vi "sing_mess.vi"(7 "Timeout(默认:5ms)":i32=5, 8 "error in":errorcluster, 9 "COM通道":u32=1, 10 "索引":i32, 11 "VISA资源名称":refnum<visa-resource-name>) -> (0 "error out 2":errorcluster, 1 "timeout":bool, 3 "VISAout":refnum<visa-resource-name>)   [LabVIEW 2012]
uses:
  com/TONGXUN/write32.vi
  com/TONGXUN/write8.vi
  <vilib>/GPower/VIRegister/VIRegister.lvlib
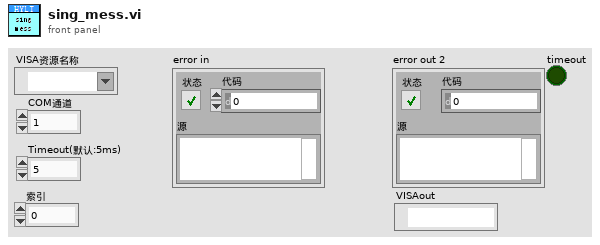
[diagram p1: front panel]
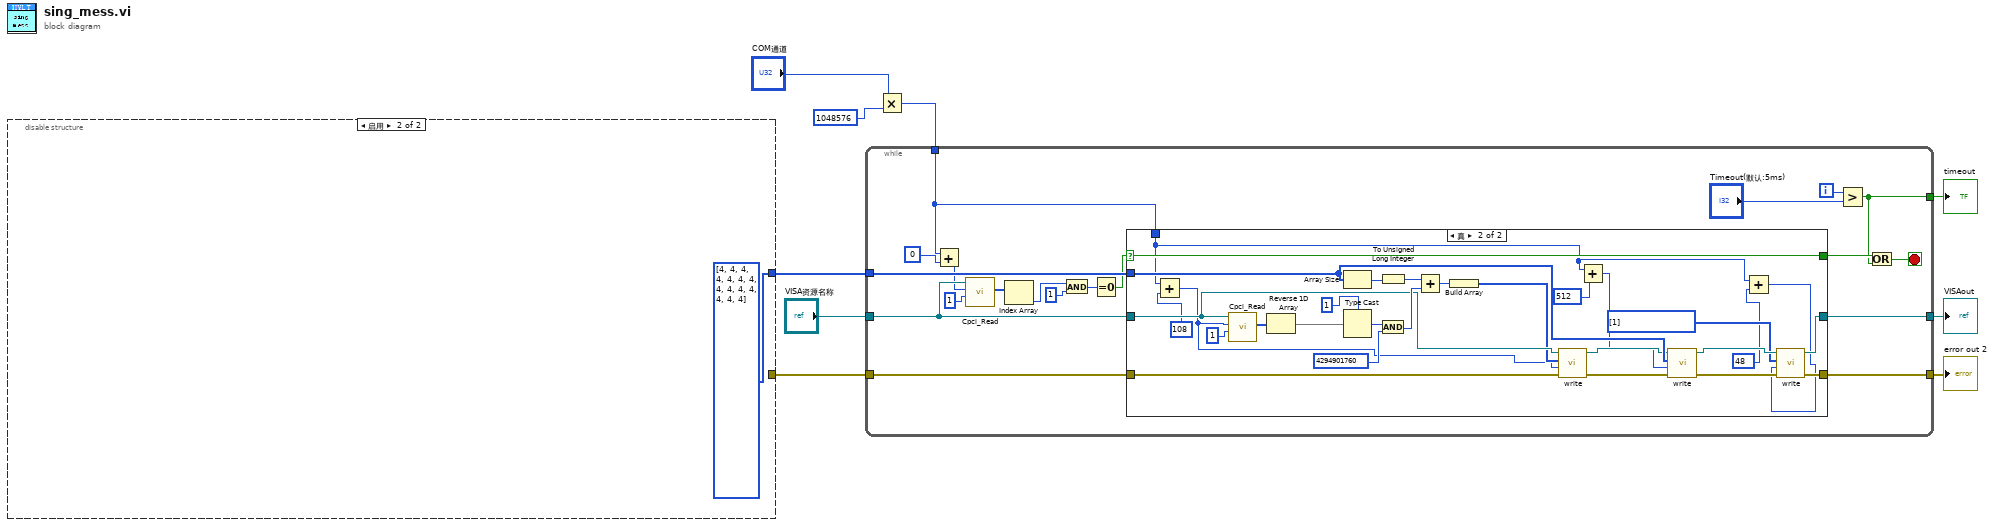
[diagram p0: block diagram]
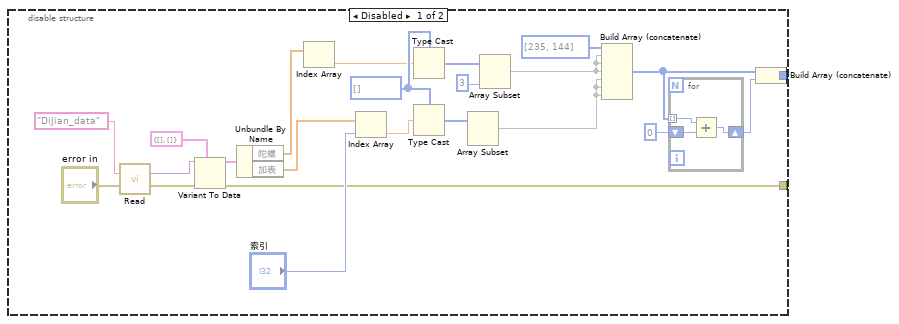
[diagram p2: hidden frame]
diagram:
  n1 = disable-structure shown="启用" {
    disable-tunnel: [w13 u8[] [4, 4, 4, 4, 4, 4, 4, 4, 4, 4, 4, 4, 4, 4]] -> w5
    disable-tunnel: [w11 _] -> w4
    frame Disabled {
      w32 = u8[] []
      n2 = call <vilib>:"Read.vi"("Register name"="DiJian_data", "Error in"="error in") -> ("Register value"=w22:variant, "Error out"=w12:errorcluster)  [unwired: 10 in, 2 out]
      n3 = Variant To Data(error in=w12, type=cluster{"陀螺":dbl[], "加表":dbl[]} {"陀螺"=[], "加表"=[]} ("输入簇"), Variant=w22) -> (data=w24:cluster{"陀螺":dbl[], "加表":dbl[]}, error out=w11:errorcluster)
      n4 = Unbundle By Name(w24) -> ("陀螺"=w25:dbl[], "加表"=w26:dbl[])
      n5 = Index Array(array=w25) -> (element=w27:dbl)  [unwired: 1 in]
      n6 = Index Array(array=w26, index="索引") -> (element=w31:dbl)
      n7 = Type Cast(type=w32, x=w27) -> (*(type *) &x=w28:u8[])
      n8 = Type Cast(type=w32, x=w31) -> (*(type *) &x=w30:u8[])
      n9 = Array Subset(array=w30) -> (w19:u8[])  [unwired: 2 in]
      n10 = Array Subset(array=w28, length=3 ("长度")) -> (w20:u8[])  [unwired: 1 in]
      n11 = Build Array (concatenate)(u8[] [235, 144] ("数组"), w20, w20, w20, w19, w19, w19) -> (w15:u8[])
      n12 = for {
        tunnel: w15 -> [w35] mode=indexing
        shift-right: [w33] -> w16
        shift-left: u8 0 ("y") -> [w34]
        n13 = Add(x=w35, y=w34) -> (x+y=w33:u8)
      }
      n14 = Build Array (concatenate)(w15, w16) -> (w13:u8[])
    }
    frame Enabled {
    }
  }
  n15 = Multiply(x="COM通道", y=u32 1048576 ("基地址")) -> (x*y=w1:u32)
  n16 = while {
    tunnel: "VISA资源名称" -> [w52]
    tunnel: w5 -> [w55]
    tunnel: w4 -> [w54]
    tunnel: [w53] -> w8
    tunnel: [w41] -> w7
    tunnel: [w40] -> w6
    tunnel: w1 -> [w37]
    i -> [w45]
    stop <- w43 stop-if-true
    n17 = Add(x=w37, y=u32 0 ("基地址")) -> (x+y=w38:u32)
    n18 = call "Cpci_Read.vi"("u32_len"=1, "基地址"=w38, "VISA资源名称"=w52) -> ("U8"=w50:u8[])  [unwired: 6 in, 2 out]
    n19 = Index Array(array=w50) -> (element=w49:u8)  [unwired: 1 in]
    n20 = And(x=w49, y=u8 1) -> (x .and. y?=w47:u8)
    n21 = Equal To 0?(x=w47) -> (x = 0?=w46:bool)
    n22 = case shown="真" w46 {
      selector: w46 -> [w58 w80]
      tunnel: w52 -> [w56 w69]
      tunnel: w55 -> [_ w87]
      tunnel: w54 -> [w57 w86]
      tunnel: [w57 w83] -> w53
      tunnel: [w58 w80] -> w42
      tunnel: [w56 w78] -> w40
      tunnel: w37 -> [_ w61]
      frame False {
      }
      frame True {
        n23 = Add(x=w61, y=u32 108 ("偏移量(0)")) -> (x+y=w64:u32)
        n24 = call "Cpci_Read.vi"("u32_len"=1, "基地址"=w64, "VISA资源名称"=w69) -> ("U8"=w73:u8[])  [unwired: 6 in, 2 out]
        n25 = Reverse 1D Array(array=w73) -> (reversed array=w74:u8[])
        n26 = Array Size(array=w87) -> (size(s)=w67:i32)
        n27 = Type Cast(type=u32 1 ("u32_len"), x=w74) -> (*(type *) &x=w76:u32)
        n28 = To Unsigned Long Integer(number=w67) -> (unsigned 32bit integer=w71:u32)
        n29 = And(x=w76, y=u32 4294901760) -> (x .and. y?=w72:u32)
        n30 = Add(x=w71, y=w72) -> (x+y=w70:u32)
        n31 = Build Array(w70) -> (w66:u32[])
        n32 = call-poly "write.vi"("error out"=w86, "起始地址"=w64, "U32"=w66, "VISA资源名称输入"=w69) -> ("error out 2"=w85:errorcluster, "VISA资源名称输出"=w79:refnum<visa-resource-name>)  [unwired: 6 in]
        n33 = Add(x=w61, y=u32 512 ("偏移量(0)")) -> (x+y=w63:u32)
        n34 = call-poly "write.vi"("error out"=w85, "起始地址"=w63, "数组"=w87, "VISA资源名称输入"=w79) -> ("error out 2"=w84:errorcluster, "VISA资源名称 输出"=w82:refnum<visa-resource-name>)  [unwired: 6 in]
        n35 = Add(x=w61, y=u32 48 ("偏移量(0)")) -> (x+y=w59:u32)
        n36 = call-poly "write.vi"("error out"=w84, "起始地址"=w59, "U32"=u32[] [1], "VISA资源名称输入"=w82) -> ("error out 2"=w83:errorcluster, "VISA资源名称输出"=w78:refnum<visa-resource-name>)  [unwired: 6 in]
      }
    }
    n37 = Greater?(x=w45, y="Timeout(默认:5ms)") -> (0:w41:bool)
    n38 = Or(x=w42, y=w41) -> (x .or. y?=w43:bool)
  }
  "error out 2" <- w8
  "timeout" <- w7
  "VISAout" <- w6
